vi "Linear Control v3.vi"(8 "Rate (unit/s)":dbl=0.2, 9 "Loop Time (ms)":u32=10, 10 "Setpoint":dbl, 11 "Recieved Motor Input":dbl) -> (2 "Currently Matching":bool, 3 "New Motor Input":dbl)   [LabVIEW 2011]
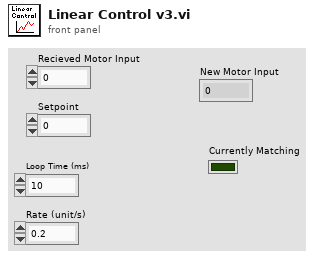
[diagram p1: front panel]
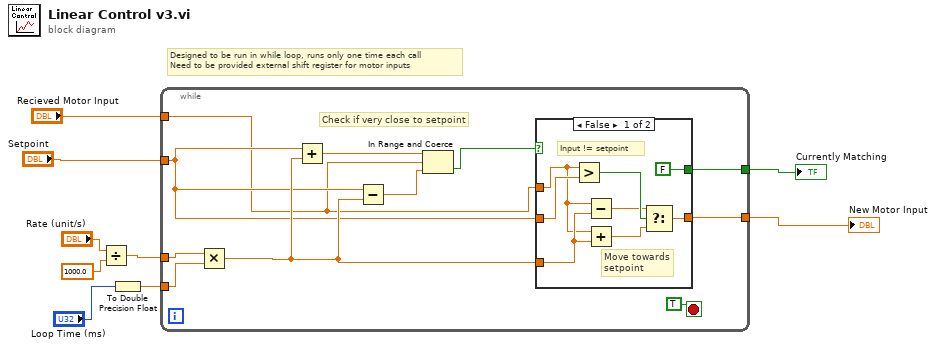
[diagram p0: block diagram]
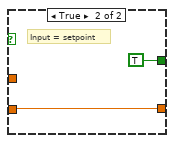
[diagram p2: hidden frame]
diagram:
  # "Designed to be run in while loop, runs only one time each call\nNeed to be provided external shift register for motor inputs"
  n1 = Divide(x="Rate (unit/s)", y=1000.0) -> (x/y=w5:dbl)
  n2 = To Double Precision Float(number="Loop Time (ms)") -> (double precision float=w1:dbl)
  n3 = while {
    tunnel: w5 -> [w17]
    tunnel: [w20] -> w9
    tunnel: [w19] -> w8
    tunnel: w1 -> [w15]
    tunnel: "Recieved Motor Input" -> [w10]
    tunnel: "Setpoint" -> [w14]
    stop <- TRUE stop-if-true
    # "Check if very close to setpoint"
    n4 = Multiply(x=w17, y=w15) -> (x*y=w16:dbl)
    n5 = Add(x=w14, y=w16) -> (x+y=w13:dbl)
    n6 = Subtract(x=w14, y=w16) -> (x-y=w12:dbl)
    n7 = In Range and Coerce(upper limit=w13, x=w10, lower limit=w12) -> (In Range?=w11:bool)  [unwired: 1 out]
    n8 = case shown="False" w11 {
      tunnel: [w23 w29] -> w19
      tunnel: w16 -> [w25 _]
      tunnel: [FALSE TRUE] -> w20
      tunnel: w14 -> [w22 w29]
      tunnel: w10 -> [w21 _]
      frame False {
        # "Move towards\nsetpoint"
        # "Input != setpoint"
        n9 = Greater?(x=w21, y=w22) -> (0:w27:bool)
        n10 = Subtract(x=w21, y=w25) -> (x-y=w26:dbl)
        n11 = Add(x=w21, y=w25) -> (x+y=w24:dbl)
        n12 = Select(t=w26, s=w27, f=w24) -> (s? t:f=w23:dbl)
      }
      frame True {
        # "Input = setpoint"
      }
    }
  }
  "Currently Matching" <- w9
  "New Motor Input" <- w8
